vi "ChangeOverGui-UpdateCounter.vi"(8 "error in":errorcluster) -> (0 "error out":errorcluster)   [LabVIEW 2016]
uses:
  ChangeOverGui.Action.ctl
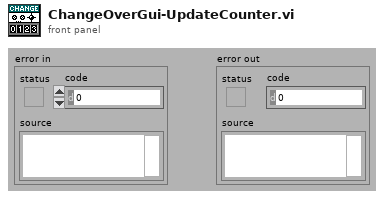
[diagram p1: front panel]
types:
  T1 = typedef "ChangeOverGui.Action.ctl" = enum32{"idle", "constructor", "destructor", "---ChangeOverGui ---", "Clear", "Validate", "Read File", "Read Imgs", "Check", "Accept", "Reject", "Scan.Begin", "Scan", "Update Table", "Update Counter", "DMC Accept"}
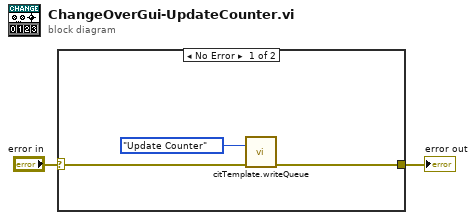
[diagram p0: block diagram]
diagram:
  n1 = case shown="No Error" "error in" {
    selector: "error in" -> [w5 w6]
    tunnel: [w3 w6] -> w1
    frame No Error {
      n2 = call "citTemplate.writeQueue.vi"("event in (if not connected:all statemachine with data event)"=ChangeOverGui.Action."Update Counter" ("Action"), "error in (no error)"=w5) -> ("error out"=w3:errorcluster)  [unwired: 13 in]
    }
    frame Error {
    }
  }
  "error out" <- w1
